vi "Read Run Parameters.vi"(8 "error in":errorcluster, 11 "TDMS in":refnum<class "TDMS.lvclass">) -> (0 "error out":errorcluster, 1 "run params":variant[](array[variant]), 2 "param names":string[](array[string]), 3 "TDMS out":refnum<class "TDMS.lvclass">)   [LabVIEW 2011, in "TDMS.lvclass"]
uses:
  TDMS.lvclass
  TDMS.lvclass/TDMS.ctl
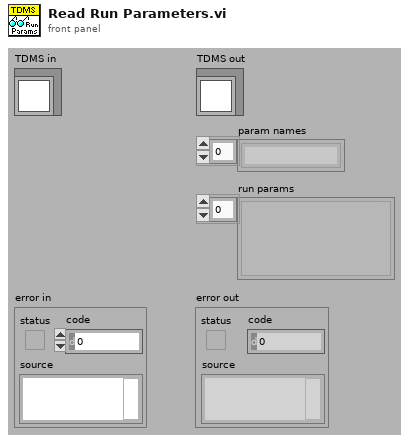
[diagram p1: front panel]
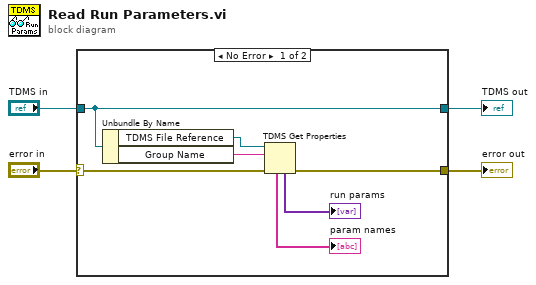
[diagram p0: block diagram]
diagram:
  n1 = case shown="No Error" "error in" {
    selector: "error in" -> [w10 w12]
    tunnel: [w9 w12] -> w1
    tunnel: [w11 w13] -> w2
    tunnel: "TDMS in" -> [w11 w13]
    frame No Error {
      n2 = Unbundle By Name(w11) -> ("TDMS File Reference"=w6:refnum<k34>, "Group Name"=w7:string)
      n3 = TDMS Get Properties(8:w10, 10:w7, 11:w6) -> (0:w9:errorcluster, 4:→"run params":variant[], 6:→"param names":string[])  [unwired: 3 in, 3 out]
    }
    frame Error {
    }
  }
  "error out" <- w1
  "TDMS out" <- w2
